vi "Joystick and Camera.vi"() -> ()   [LabVIEW 2021]
uses:
  Classes/Controller/Camera/Machine Vision.ctl
  Classes/Controller/Camera/Image processing.ctl
  Classes/Controller/Camera/Camera settings.ctl
  Classes/Controller/Camera/Material.ctl
  Classes/Controller/I-O/I-O.lvclass
  Classes/Controller/Camera/Camera.lvclass
  Classes/Controller/Controller.lvclass
  Classes/Controller/Motion/A3200/A3200.lvclass
  Classes/Controller/Motion/Motion.lvclass
  <vilib>/vision/driver/NI_Vision_Acquisition_Software.lvlib
panel:
  out "Move by":dbl[](array[numeric])
  in  "Autofiducial":bool
  in  "Screen Grab":bool
  in  "Focus step size":dbl format="%#_13g"
  in  "number of focus steps":i32
  out "Radius (Real-World)":dbl
  out "error out":errorcluster
  in  "Find fiducial center":bool
  out "Average Strength":dbl
  in  "Focus":bool
  in  "Material":T1
  in  "Override presets":bool
  in  "Camera settings":T2={"Gamma"=1.6, "Gain"=0, "Sharpness"=0, "Contrast"=0.0, "Exposure"=0.0078125} {"Exposure" min=0.000244140625 max=0.5 scale=0.0002..0.5; "Contrast" min=0.0 max=1.0 scale=0.0..1.0; "Sharpness" min=0 max=2 step=1 scale=0.0..2.0; "Gain" min=0 max=100 step=1 scale=0.0..100.0; "Gamma" min=0.01 max=10.0 scale=0.01..10.0}
  in  "Image processing":T3={"Brightness"=128.0, "Contrast"=45.0, "Gamma"=1.0471123} {"Brightness" scale=0.0..400.0; "Contrast" scale=0.0..90.0; "Gamma" scale=0.005..5.0}
  out "XYZTheta Out":dbl[](array[numeric])
  in  "Machine Vision":T4
  in  "Move 10cm Right":bool
  in  "Move 10cm Backward":bool
  in  "Move 10cm Forward":bool
  in  "Move 10cm Left":bool
  in  "Record Measurement":bool=TRUE
  in  "Dismount Silicon Tray":bool
  in  "Secure Silicon Tray":bool
  in  "Z Go":bool
  in  "Position":dbl
  in  "XYZTheta":dbl[](array[numeric])
  in  "Go":bool
  in  "Joystick":bool
  out "Sum":dbl[](array[numeric]) format="%#.6g"
  out "Gantry":dbl[](array[numeric]) format="%#.6g"
  in  "Stop":bool
  out "Image":T5(plugin-control)
  out "Camera":dbl[](array[numeric])
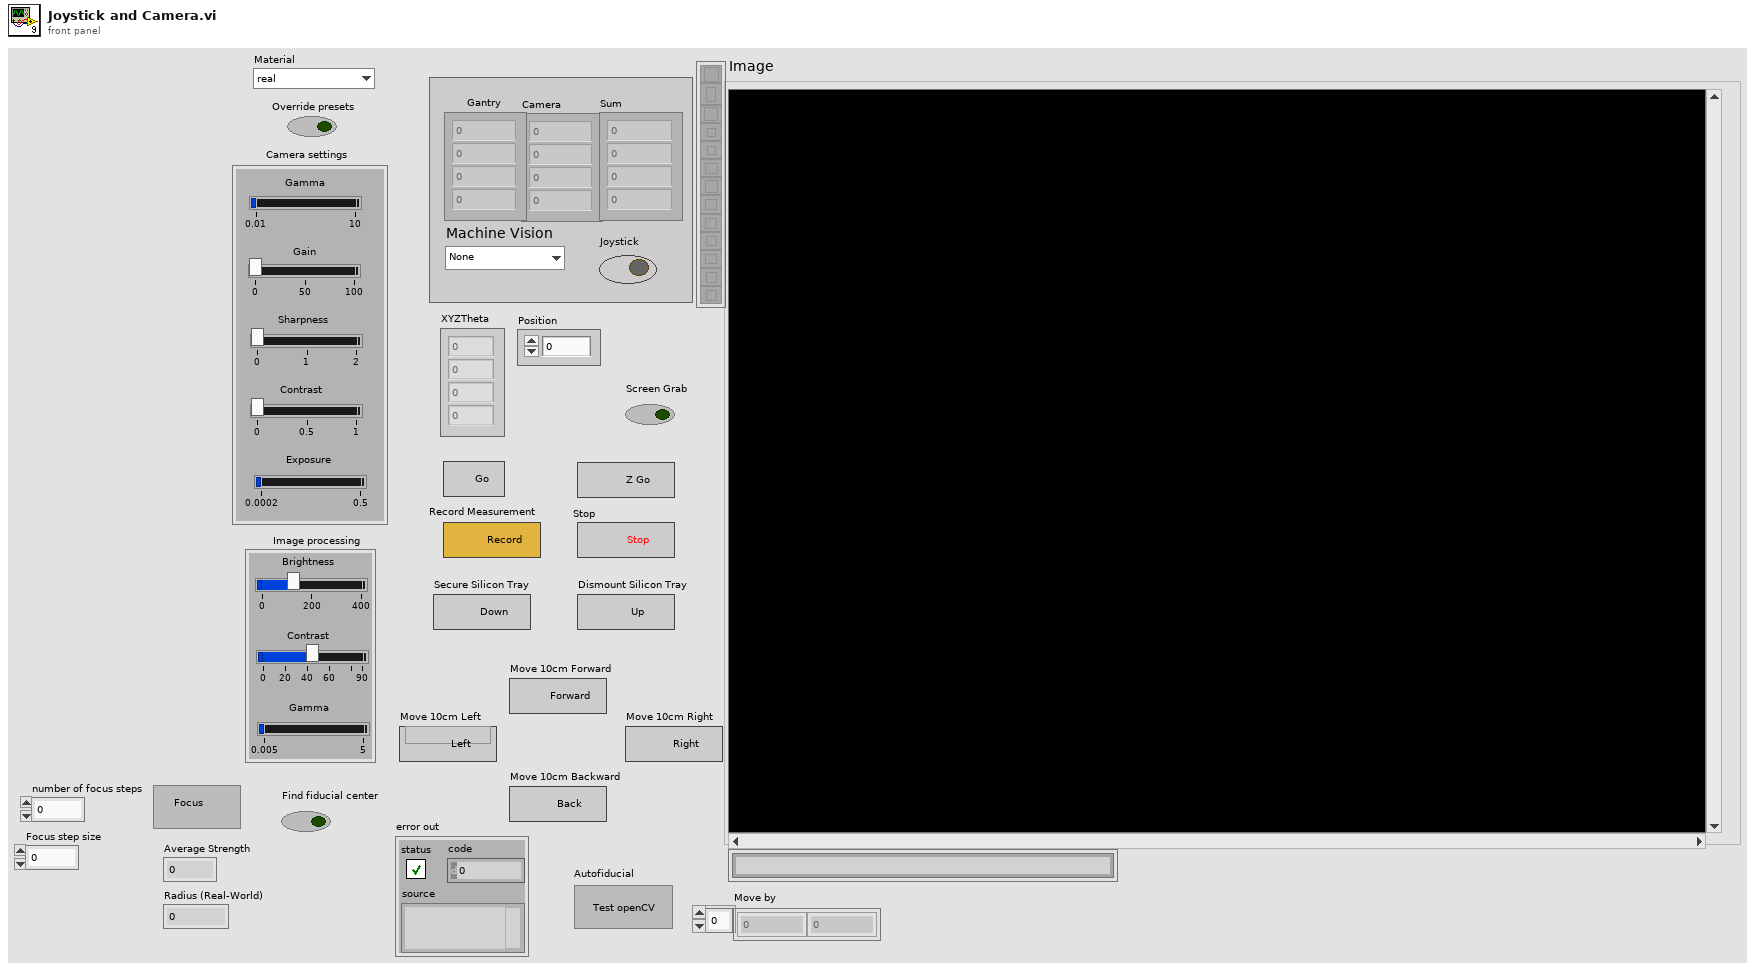
[diagram p1: front panel]
types:
  T1 = typedef "Camera.lvclass/Material.ctl" = enum16{"real", "dummy", "PETG"}
  T2 = typedef "Camera.lvclass/Camera settings.ctl" = cluster{"Gamma":dbl, "Gain":i64, "Sharpness":i64, "Contrast":dbl, "Exposure":dbl}
  T3 = typedef "Camera.lvclass/Image processing.ctl" = cluster{"Brightness":sgl, "Contrast":sgl, "Gamma":sgl}
  T4 = typedef "Camera.lvclass/Machine Vision.ctl" = enum16{"None", "Tray Fiducials", "HPK Silicon", "100um dot", "Hexaboard", "Corner (TL, BR)", "Corner (BL, TR)", "BP gold pad 1", "BP gold pad 2", "BP gold pad 3", "dummy sensor CH2", "dummy sensor CH7", "dummy sensor CH191", "dummy sensor CH197", "sensor circle", "sensor cross"}
  T5 = typedef "IMAQ Image.ctl" = refnum<image>
  T6 = enum16{"open", "replace", "create", "open or create", "replace or create", "replace or create with confirmation"}
  T7 = typedef "Controller.lvclass/Controllers.ctl" = cluster{"I-O.lvclass":refnum<class "I-O.lvclass">, "Gantry":refnum<k24>, "Dispenser":refnum<visa-resource-name>}
  T8 = typedef "I-O.lvclass/Pin Map.ctl" = cluster{"Region Valves":i32[], "Extra Valves":dbl[][][], "Tool Primary Valve":i32, "Tool Secondary Valve":i32, "Region Sensors":i32[], "Extra Sensors":dbl[][][], "Tool Primary Sensor":dbl, "Tool Secondary Sensor":dbl, "Compression Sensor":dbl, "5V":i32, "Dispenser Sensor":dbl}
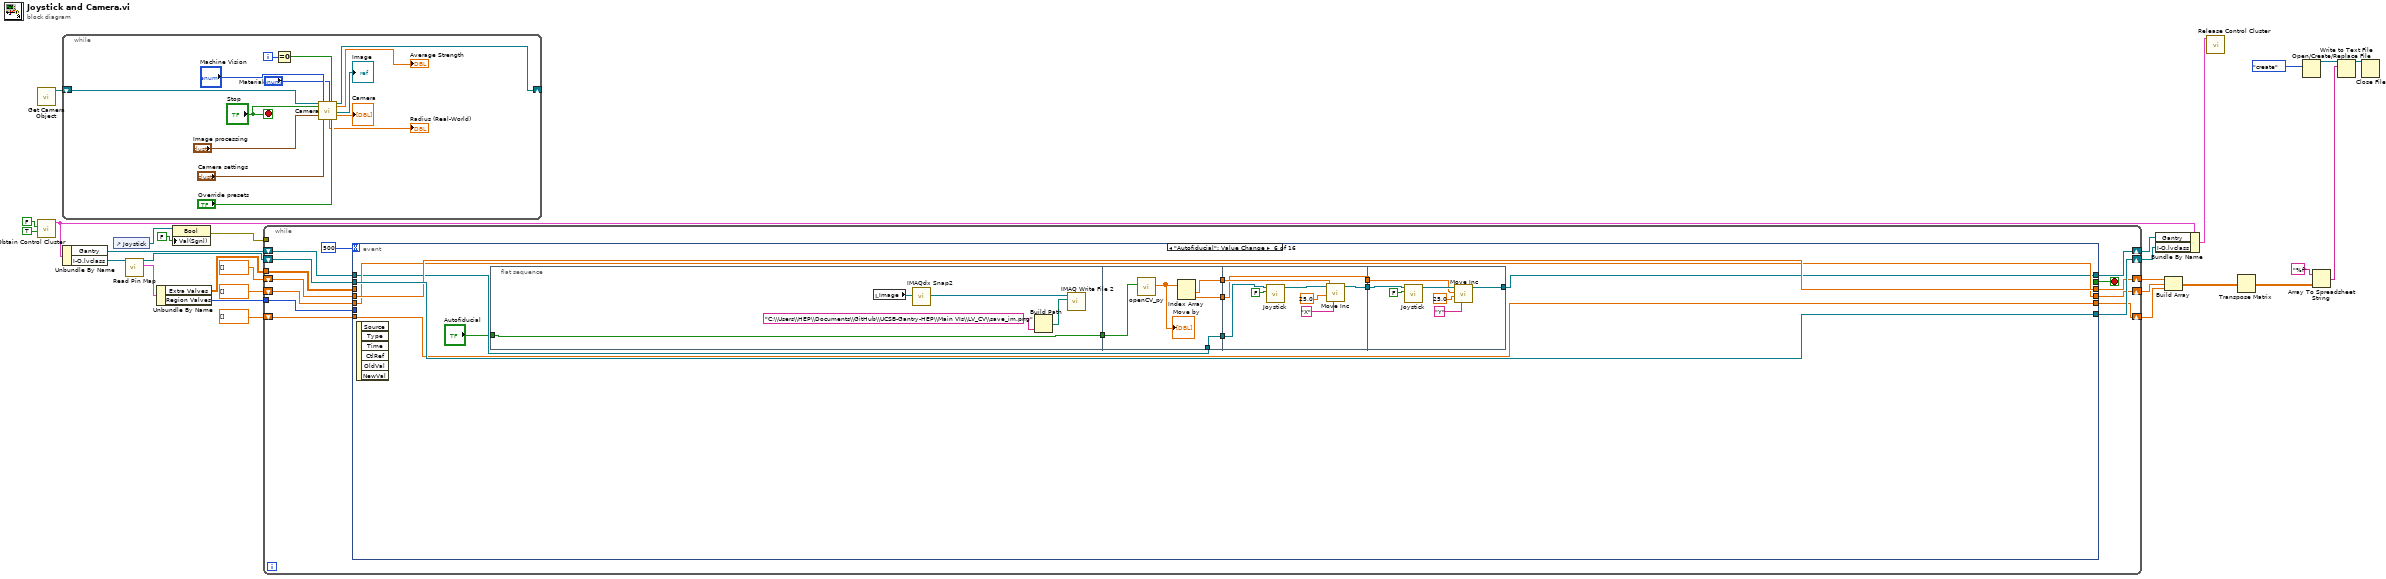
[diagram p0: block diagram]
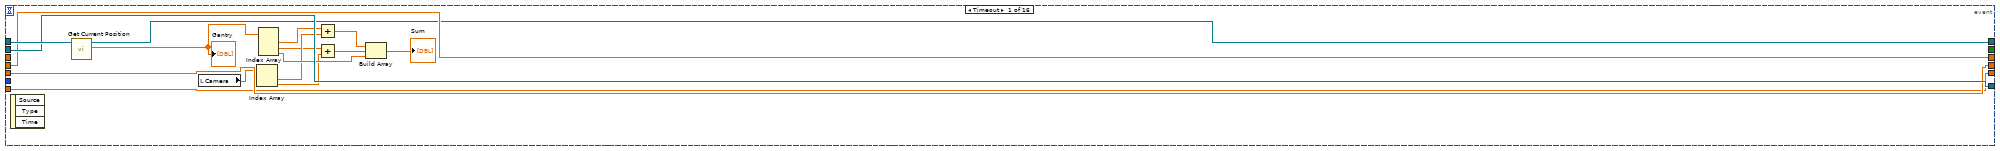
[diagram p2: hidden frame]
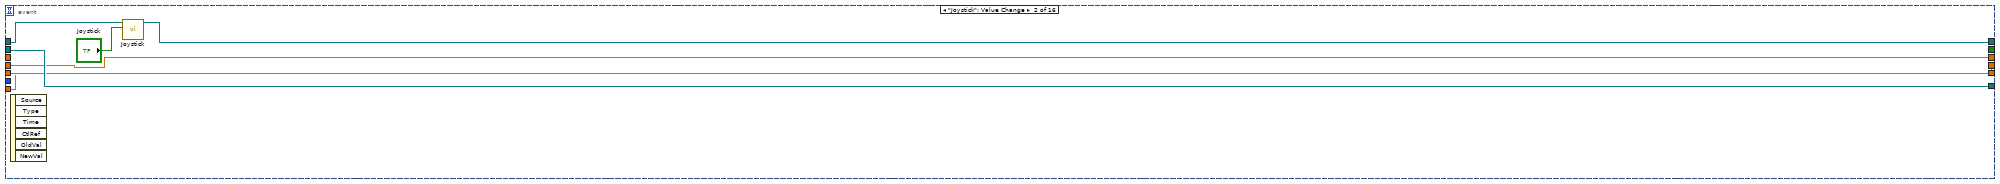
[diagram p3: hidden frame]
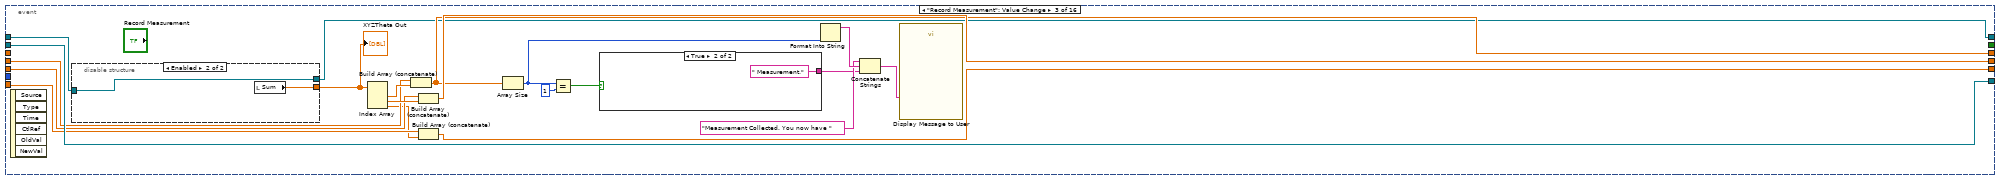
[diagram p4: hidden frame]
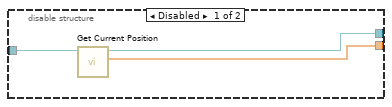
[diagram p5: hidden frame]
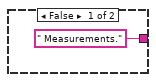
[diagram p6: hidden frame]
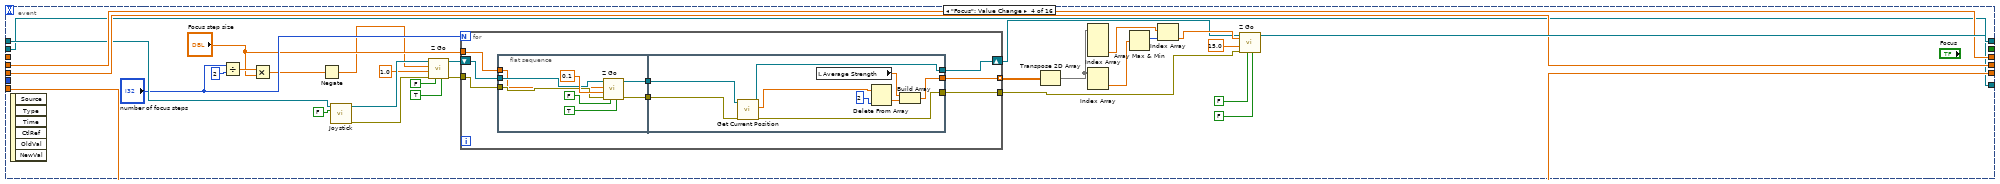
[diagram p7: hidden frame]
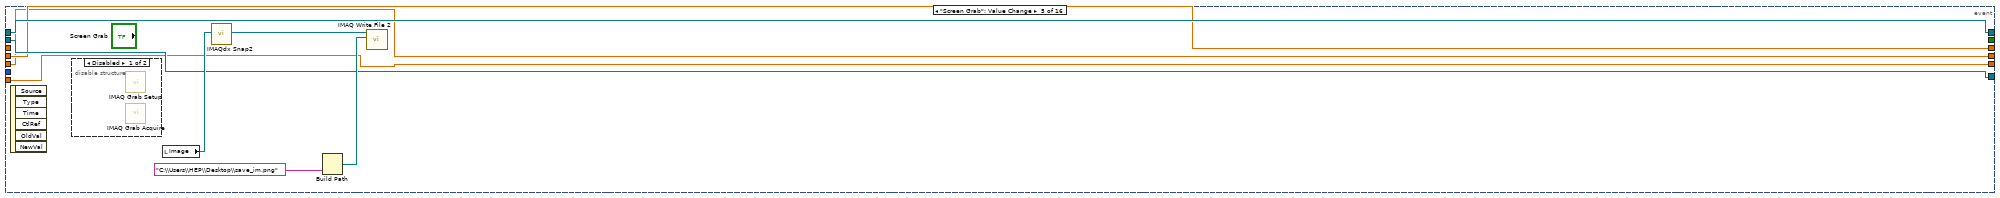
[diagram p8: hidden frame]
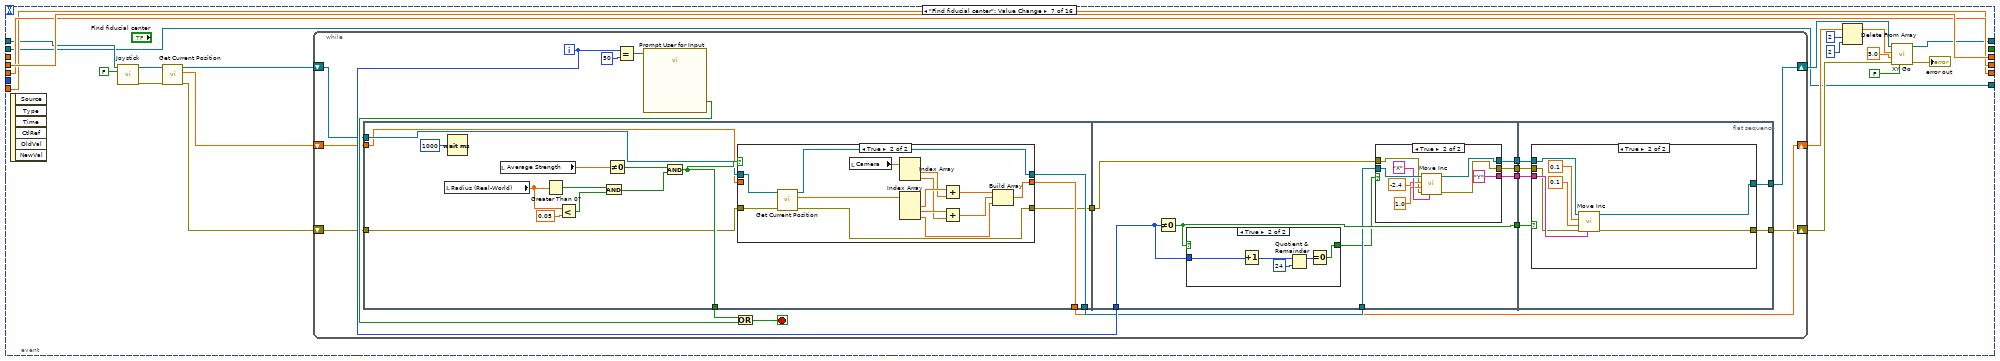
[diagram p10: hidden frame]
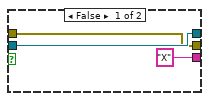
[diagram p13: hidden frame]
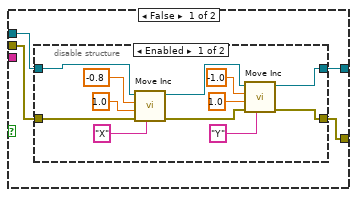
[diagram p14: hidden frame]
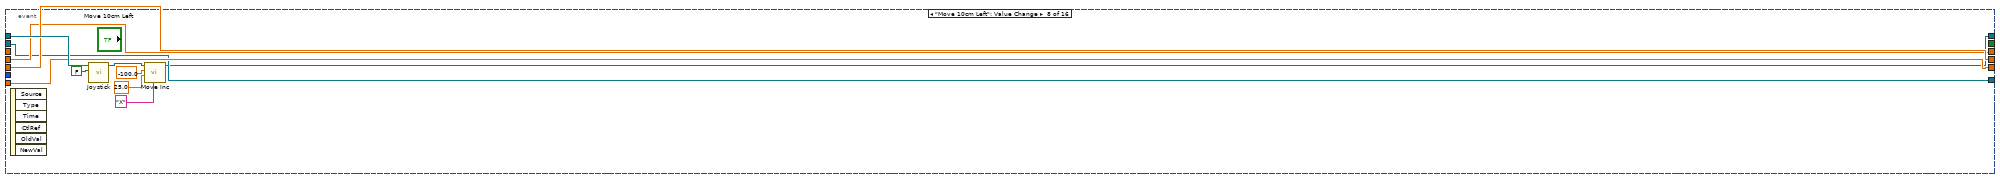
[diagram p16: hidden frame]
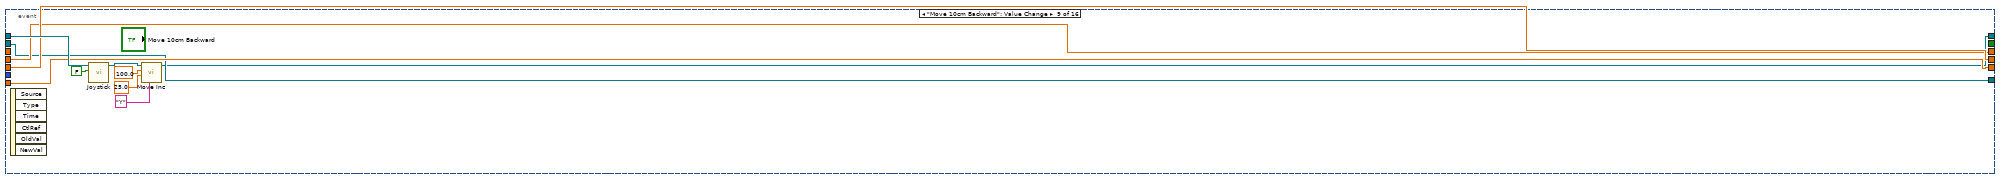
[diagram p17: hidden frame]
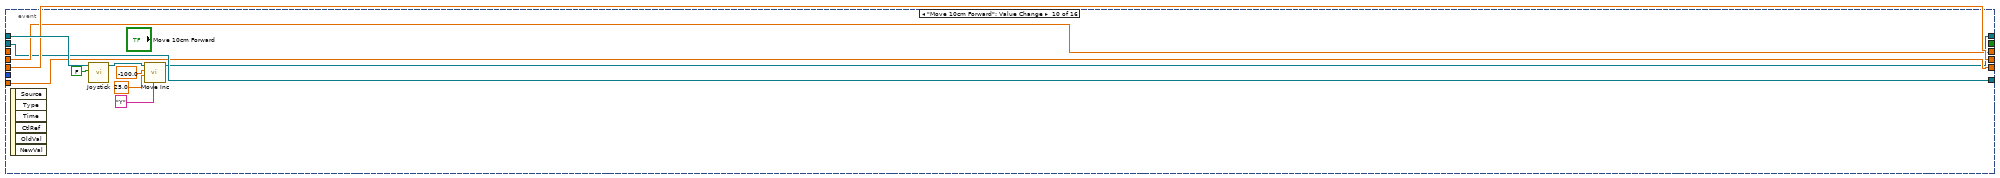
[diagram p18: hidden frame]
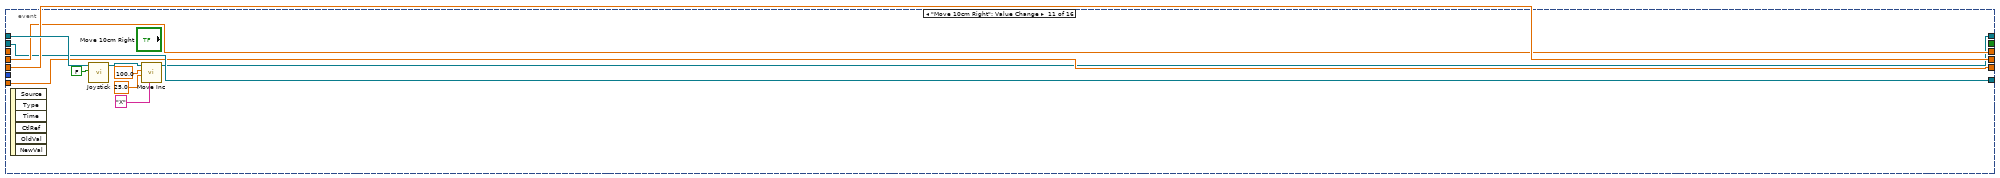
[diagram p19: hidden frame]
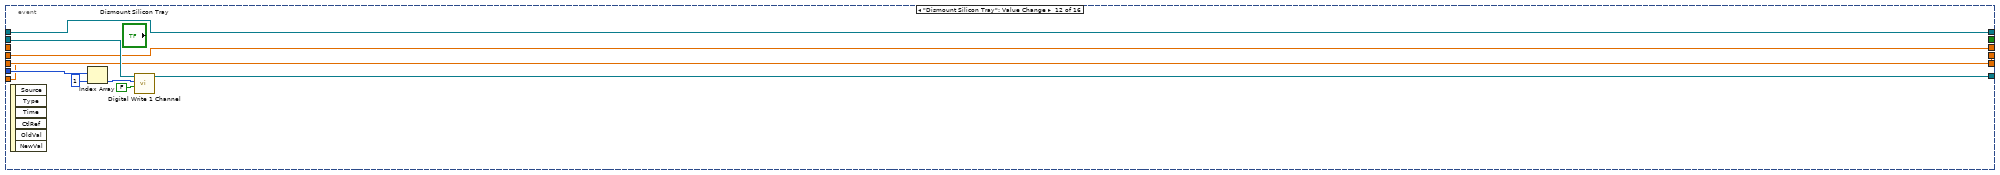
[diagram p20: hidden frame]
diagram:
  n1 = call "Get Camera Object.vi"() -> ("Camera out"=w23:refnum<class "Camera.lvclass">)  [unwired: 10 in, 1 out]
  n2 = call "Obtain Control Cluster.vi"("I/O"=TRUE, "Dispense"=FALSE) -> ("Control Out"=w1:T7)  [unwired: 9 in]
  n3 = while {
    shift-right: [w42] -> _
    shift-left: w23 -> [w43]
    i -> [w34]
    stop <- "Stop" stop-if-true
    n4 = Equal To 0?(x=w34) -> (x = 0?=w33:bool)
    n5 = call "Camera.vi"("Camera in"=w43, "Stop"="Stop", "BCG Image Processing"="Image processing", "Machine Vision"="Machine Vision", "Camera settings"="Camera settings", "Material"="Material", "Loop 0"=w33, "Override presets"="Override presets") -> ("Radius (Real-World)"=→"Radius (Real-World)":dbl, "Camera out"=w42:refnum<class "Camera.lvclass">, "Average Strength"=→"Average Strength":dbl, "Image"=→"Image":T5, "Camera"=→"Camera":dbl[])  [unwired: 6 in, 1 out]
  }
  n6 = Unbundle By Name(w1) -> ("Gantry"=w24:refnum<k24>, "I-O.lvclass"=w22:refnum<class "I-O.lvclass">)
  n7 = control-ref of="Joystick"() -> (w28:refnum<vi>)
  n8 = call-dynamic "Read Pin Map.vi"("I-O in"=w22) -> ("Pin Map 2"=w20:T8, "I-O out"=w21:refnum<class "I-O.lvclass">)  [unwired: 8 in, 1 out]
  n9 = Unbundle By Name(w20) -> ("Extra Valves"=w18:dbl[][][], "Region Valves"=w19:i32[])
  n10 = property class="Bool"(reference=w28, "Val(Sgnl)"=FALSE ("Value (Signaling)")) -> (error out=w27:errorcluster)  [unwired: 1 in, 1 out]
  n11 = while {
    shift-right: [w44] -> w4
    shift-left: w24 -> [w55]
    tunnel: w27 -> [_]
    shift-right: [w53] -> w3
    shift-left: w21 -> [w54]
    tunnel: w19 -> [w52]
    tunnel: w18 -> [w51]
    shift-right: [w46] -> w6
    shift-left: dbl[] [] -> [w50]
    shift-right: [w48] -> w7
    shift-left: dbl[] [] -> [w49]
    shift-right: [w45] -> w8
    shift-left: dbl[] [] -> [w47]
    stop <- w56 stop-if-true
    n12 = event shown="[5] \"Autofiducial\": Value Change" {
      selector: _ -> [_ _ _ _ _ _ _ _ _ _ _ _ _ _ _ _]
      dyn-events: _ -> [_ _ _ _ _ _ _ _ _ _ _ _ _ _ _ _]
      timeout: 500 -> [_ _ _ _ _ _ _ _ _ _ _ _ _ _ _ _]
      tunnel: [_ _ _ _ _ _ _ _ _ _ _ _ _ _ _ TRUE] -> w56
      tunnel: w55 -> [w73 w80 w83 w124 w168 w180 w228 w347 w358 w369 w380 w382 w392 w409 w428 w436]
      tunnel: w54 -> [w72 w78 w100 w108 w167 w185 w211 w342 w354 w366 w377 w389 w401 w406 w425 w434]
      tunnel: [w72 w78 w100 w108 w167 w185 w211 w342 w354 w366 w377 w386 w396 w406 w425 w434] -> w53
      tunnel: w52 -> [_ _ _ _ _ _ _ _ _ _ _ w391 w400 _ _ _]
      tunnel: w51 -> [_ _ _ _ _ _ _ _ _ _ _ _ _ _ _ _]
      tunnel: w50 -> [w71 w77 w87 w127 w165 w183 w230 w345 w357 w368 w379 w385 w395 w405 w424 w433]
      tunnel: [w71 w77 w91 w127 w165 w183 w230 w345 w357 w368 w379 w385 w395 w405 w424 w433] -> w46
      tunnel: w49 -> [w70 w76 w88 w128 w166 w184 w231 w344 w356 w367 w378 w384 w394 w404 w423 w432]
      tunnel: [w70 w76 w90 w128 w166 w184 w231 w344 w356 w367 w378 w384 w394 w404 w423 w432] -> w48
      tunnel: w47 -> [w69 w75 w86 w126 w164 w182 w229 w343 w355 w365 w376 w383 w393 w403 w422 w431]
      tunnel: [w69 w75 w84 w126 w164 w182 w229 w343 w355 w365 w376 w383 w393 w403 w422 w431] -> w45
      tunnel: [w68 w74 w81 w129 w168 w179 w225 w341 w350 w360 w372 w382 w392 w402 w421 w429] -> w44
      event Timeout {
        n13 = event-data() -> ()  [unwired: 1 in, 3 out]
        n14 = call "Get Current Position.vi"("Gantry In"=w73) -> ("XYZTheta Out"=w65:dbl[], "Gantry Out"=w68:refnum<k24>)  [unwired: 8 in, 1 out]
        "Gantry" <- w65
        n15 = local read "Camera"() -> (w62:dbl[])
        n16 = Index Array(array=w62) -> (element #1=w61:dbl, element #2=w58:dbl)  [unwired: 2 in]
        n17 = Index Array(array=w65) -> (element #1=w63:dbl, element #2=w59:dbl, element #3=w66:dbl)  [unwired: 3 in]
        n18 = Add(x=w63, y=w61) -> (x+y=w64:dbl)
        n19 = Add(x=w59, y=w58) -> (x+y=w60:dbl)
        n20 = Build Array(w64, w60, w66) -> (→"Sum":dbl[])
      }
      event "Joystick": Value Change {
        n21 = event-data() -> ()  [unwired: 1 in, 6 out]
        n22 = call "Joystick.vi"("Joystick"="Joystick", "Gantry In"=w80) -> ("Gantry Out"=w74:refnum<k24>)  [unwired: 8 in, 1 out]
      }
      event "Record Measurement": Value Change {
        n23 = event-data() -> ()  [unwired: 1 in, 6 out]
        n24 = disable-structure shown="Enabled" {
          disable-tunnel: [w102 w104] -> w82
          disable-tunnel: w83 -> [w103 w105]
          disable-tunnel: [w101 w105] -> w81
          frame Disabled {
            n25 = call "Get Current Position.vi"("Gantry In"=w103) -> ("XYZTheta Out"=w102:dbl[], "Gantry Out"=w101:refnum<k24>)  [unwired: 8 in, 1 out]
          }
          frame Enabled {
            n26 = local read "Sum"() -> (w104:dbl[])
          }
        }
        "XYZTheta Out" <- w82
        n27 = Index Array(array=w82) -> (element #1=w99:dbl, element #2=w89:dbl, element #3=w85:dbl)  [unwired: 3 in]
        n28 = Build Array (concatenate) "Build Array"(w88, w99) -> (w90:dbl[])
        n29 = Build Array (concatenate)(w87, w89) -> (w91:dbl[])
        n30 = Build Array (concatenate)(w86, w85) -> (w84:dbl[])
        n31 = Array Size(array=w90) -> (size(s)=w94:i32)
        n32 = Equal?(x=w94, y=1) -> (x = y?=w93:bool)
        n33 = case shown="True" w93 {
          tunnel: [" Measurements." " Measurement."] -> w92
          frame False {
          }
          frame True {
          }
        }
        n34 = Format Into String(w94) -> (resulting string=w98:string)  [unwired: 3 in, 1 out]
        n35 = Concatenate Strings("Measurement Collected. You now have ", w98, w92) -> (w96:string)
        n36 = call "Display Message to User"("Message"=w96) -> ()  [unwired: 9 in, 2 out]
      }
      event "Focus": Value Change {
        n37 = event-data() -> ()  [unwired: 1 in, 6 out]
        n38 = Divide(x="number of focus steps", y=2) -> (x/y=w121:dbl)
        n39 = Multiply(x=w121, y="Focus step size") -> (x*y=w119:dbl)
        n40 = Negate(x=w119) -> (-x=w114:dbl)
        n41 = call "Joystick.vi"("Joystick"=FALSE, "Gantry In"=w124) -> ("error out"=w115:errorcluster, "Gantry Out"=w118:refnum<k24>)  [unwired: 8 in]
        n42 = call "Z Go.vi"("Increment"=TRUE, "Return Immediately"=FALSE ("Increment"), "error in (no error)"=w115, "Speed In"=1.0 ("Speed"), "Position In"=w114, "Gantry In"=w118) -> ("error out"=w116:errorcluster, "Gantry Out"=w117:refnum<k24>)  [unwired: 2 in, 2 out]
        n43 = for {
          N: "number of focus steps" -> [_]
          tunnel: [w143] -> w137 mode=indexing
          tunnel: w116 -> [w142]
          tunnel: [w140] -> w130
          shift-right: [w144] -> w131
          shift-left: w117 -> [w146]
          tunnel: "Focus step size" -> [w139]
          n44 = flat-sequence {
            tunnel: w146 -> [w153]
            tunnel: [w152] -> w145
            tunnel: w142 -> [w151]
            tunnel: [w150] -> w141
            tunnel: w139 -> [w149]
            tunnel: w145 -> [w163]
            tunnel: [w162] -> w144
            tunnel: [w161] -> w143
            tunnel: w141 -> [w157]
            tunnel: [w156] -> w140
            frame #0 {
              n45 = call "Z Go.vi"("Increment"=TRUE, "Return Immediately"=FALSE ("Increment"), "error in (no error)"=w151, "Speed In"=0.1 ("Speed"), "Position In"=w149, "Gantry In"=w153) -> ("error out"=w150:errorcluster, "Gantry Out"=w152:refnum<k24>)  [unwired: 2 in, 2 out]
            }
            frame #1 {
              n46 = call "Get Current Position.vi"("error in (no error)"=w157, "Gantry In"=w163) -> ("error out"=w156:errorcluster, "XYZTheta Out"=w160:dbl[], "Gantry Out"=w162:refnum<k24>)  [unwired: 7 in]
              n47 = local read "Average Strength"() -> (w155:dbl)
              n48 = Delete From Array(array=w160, index=2) -> (deleted portion=w158:dbl)  [unwired: 1 in, 1 out]
              n49 = Build Array(w155, w158) -> (w161:dbl[])
            }
          }
        }
        n50 = Transpose 2D Array(2D array=w137) -> (transposed array=w136:dbl[][])
        n51 = Index Array(array=w136) -> (element #2=w135:dbl[])  [unwired: 4 in, 1 out]
        n52 = Index Array(array=w136) -> (element=w138:dbl[])  [unwired: 2 in]
        n53 = Array Max & Min(array=w138) -> (max index (indices)=w134:i32)  [unwired: 3 out]
        n54 = Index Array(array=w135, index=w134) -> (element=w133:dbl)
        n55 = call "Z Go.vi"("Increment"=FALSE, "Return Immediately"=FALSE ("Increment"), "error in (no error)"=w130, "Speed In"=15.0 ("Speed"), "Position In"=w133, "Gantry In"=w131) -> ("Gantry Out"=w129:refnum<k24>)  [unwired: 2 in, 3 out]
      }
      event "Screen Grab": Value Change {
        n56 = event-data() -> ()  [unwired: 1 in, 6 out]
        n57 = disable-structure shown="Disabled" {
          frame Disabled {
            n58 = call <vilib>:"IMAQ Grab Setup.vi"() -> ()  [unwired: 10 in, 2 out]
            n59 = call <vilib>:"IMAQ Grab Acquire.vi"() -> ()  [unwired: 8 in, 4 out]
          }
          frame Enabled {
          }
        }
        n60 = local read "Image"() -> (w172:T5)
        n61 = call <vilib>:"IMAQdx Snap2.vi"("Image In"=w172) -> ("Image Out"=w171:T5)  [unwired: 8 in, 2 out]
        n62 = Build Path(name or relative path="C:\\Users\\HEP\\Desktop\\save_im.png") -> (appended path=w170:path)  [unwired: 1 in]
        n63 = call-poly "IMAQ Write File 2"("File Path"=w170, "Image"=w171) -> ()  [unwired: 8 in, 2 out]
      }
      event "Autofiducial": Value Change {
        n64 = event-data() -> ()  [unwired: 1 in, 6 out]
        n65 = flat-sequence {
          tunnel: [w186] -> w181
          tunnel: "Autofiducial" -> [w186]
          tunnel: w181 -> [w195]
          tunnel: w180 -> [w194]
          tunnel: [w194] -> w177
          tunnel: [w192] -> w175
          tunnel: [w191] -> w173
          tunnel: w177 -> [w199]
          tunnel: [w198] -> w176
          tunnel: w175 -> [w197]
          tunnel: [w196] -> w174
          tunnel: w173 -> [w196]
          tunnel: [w205] -> w179
          tunnel: w176 -> [w206]
          tunnel: w174 -> [w204]
          frame #0 {
            n66 = local read "Image"() -> (w190:T5)
            n67 = call <vilib>:"IMAQdx Snap2.vi"("Image In"=w190) -> ("Image Out"=w189:T5)  [unwired: 8 in, 2 out]
            n68 = Build Path(name or relative path="C:\\Users\\HEP\\Documents\\GitHub\\UCSB-Gantry-HEP\\Main VIs\\LV_CV\\save_im.png") -> (appended path=w188:path)  [unwired: 1 in]
            n69 = call-poly "IMAQ Write File 2"("File Path"=w188, "Image"=w189) -> ()  [unwired: 8 in, 2 out]
          }
          frame #1 {
            n70 = call "openCV_py.vi"("Run PY"=w195) -> ("Move by"=w193:dbl[])  [unwired: 10 in]
            "Move by" <- w193
            n71 = Index Array(array=w193) -> (element #1=w192:dbl, element #2=w191:dbl)  [unwired: 2 in]
          }
          frame #2 {
            n72 = call "Joystick.vi"("Joystick"=FALSE, "Gantry In"=w199) -> ("Gantry Out"=w200:refnum<k24>)  [unwired: 8 in, 1 out]
            n73 = call "Move Inc.vi"("Axis"="X", "Speed"=25.0, "Distance"=w197, "Gantry In"=w200) -> ("Gantry Out"=w198:refnum<k24>)  [unwired: 6 in, 1 out]
          }
          frame #3 {
            n74 = call "Joystick.vi"("Joystick"=FALSE, "Gantry In"=w206) -> ("Gantry Out"=w207:refnum<k24>)  [unwired: 8 in, 1 out]
            n75 = call "Move Inc.vi"("Axis"="Y", "Speed"=25.0, "Distance"=w204, "Gantry In"=w207) -> ("Gantry Out"=w205:refnum<k24>)  [unwired: 6 in, 1 out]
          }
        }
      }
      event "Find fiducial center": Value Change {
        n76 = event-data() -> ()  [unwired: 1 in, 6 out]
        n77 = call "Joystick.vi"("Joystick"=FALSE, "Gantry In"=w228) -> ("error out"=w217:errorcluster, "Gantry Out"=w219:refnum<k24>)  [unwired: 8 in]
        n78 = call "Get Current Position.vi"("error in (no error)"=w217, "Gantry In"=w219) -> ("error out"=w216:errorcluster, "XYZTheta Out"=w214:dbl[], "Gantry Out"=w218:refnum<k24>)  [unwired: 7 in]
        n79 = while {
          shift-right: [w248] -> w226
          shift-left: w218 -> [w237]
          shift-right: [w249] -> w224
          shift-left: w216 -> [w234]
          shift-right: [w232] -> w213
          shift-left: w214 -> [w235]
          i -> [w243]
          stop <- w241 stop-if-true
          n80 = flat-sequence {
            tunnel: [w261] -> w238
            tunnel: [w260] -> w232
            tunnel: w237 -> [w259]
            tunnel: [w258] -> w236
            tunnel: w235 -> [w257]
            tunnel: w234 -> [w256]
            tunnel: [w255] -> w233
            tunnel: w243 -> [w289]
            tunnel: [w288] -> w247
            tunnel: [w287] -> w246
            tunnel: w236 -> [w286]
            tunnel: [w285] -> w245
            tunnel: [w284] -> w244
            tunnel: w233 -> [w282]
            tunnel: [w310] -> w248
            tunnel: [w311] -> w249
            tunnel: w247 -> [w312]
            tunnel: w246 -> [w309]
            tunnel: w245 -> [w308]
            tunnel: w244 -> [w307]
            frame #0 {
              n81 = local read "Radius (Real-World)"() -> (w251:dbl)
              n82 = Wait (ms)(milliseconds to wait=u32 1000) -> ()  [unwired: 1 out]
              n83 = local read "Average Strength"() -> (w264:dbl)
              n84 = Greater Than 0?(x=w251) -> (x > 0?=w253:bool)
              n85 = Less?(x=w251, y=0.05) -> (x < y?=w252:bool)
              n86 = And(x=w253, y=w252) -> (x .and. y?=w262:bool)
              n87 = Not Equal To 0?(x=w264) -> (x != 0?=w263:bool)
              n88 = And(x=w263, y=w262) -> (x .and. y?=w261:bool)
              n89 = case shown="True" w261 {
                tunnel: [w266 w270] -> w260
                tunnel: w259 -> [w267 w281]
                tunnel: [w267 w280] -> w258
                tunnel: w257 -> [w266 _]
                tunnel: w256 -> [w265 w269]
                tunnel: [w265 w268] -> w255
                frame False {
                }
                frame True {
                  n90 = call "Get Current Position.vi"("error in (no error)"=w269, "Gantry In"=w281) -> ("error out"=w268:errorcluster, "XYZTheta Out"=w279:dbl[], "Gantry Out"=w280:refnum<k24>)  [unwired: 7 in]
                  n91 = local read "Camera"() -> (w277:dbl[])
                  n92 = Index Array(array=w277) -> (element #1=w274:dbl, element #2=w273:dbl)  [unwired: 2 in]
                  n93 = Index Array(array=w279) -> (element #1=w278:dbl, element #2=w275:dbl, element #3=w276:dbl)  [unwired: 3 in]
                  n94 = Add(x=w278, y=w274) -> (x+y=w272:dbl)
                  n95 = Add(x=w275, y=w273) -> (x+y=w271:dbl)
                  n96 = Build Array(w272, w271, w276) -> (w270:dbl[])
                }
              }
            }
            frame #1 {
              n97 = Not Equal To 0?(x=w289) -> (x != 0?=w287:bool)
              n98 = case shown="True" w287 {
                selector: w287 -> [w290 _]
                tunnel: [w290 w294] -> w283
                tunnel: w289 -> [_ w292]
                frame False {
                }
                frame True {
                  n99 = Increment(x=w292) -> (x+1=w291:i32)
                  n100 = Quotient & Remainder(x=w291, y=24) -> (x-y*floor(x/y)=w293:i32)  [unwired: 1 out]
                  n101 = Equal To 0?(x=w293) -> (x = 0?=w294:bool)
                }
              }
              n102 = case shown="True" w283 {
                tunnel: ["X" ("Axis") "Y" ("Axis")] -> w288
                tunnel: w286 -> [w297 w305]
                tunnel: [w297 w304] -> w285
                tunnel: [w296 w300] -> w284
                tunnel: w282 -> [w296 w299]
                frame False {
                }
                frame True {
                  n103 = call "Move Inc.vi"("Axis"="X", "error in (no error)"=w299, "Speed"=1.0, "Distance"=-2.4, "Gantry In"=w305) -> ("error out"=w300:errorcluster, "Gantry Out"=w304:refnum<k24>)  [unwired: 5 in]
                }
              }
            }
            frame #2 {
              n104 = case shown="True" w309 {
                tunnel: w312 -> [_ w337]
                tunnel: w307 -> [w313 w336]
                tunnel: w308 -> [w316 w334]
                tunnel: [w314 w333] -> w311
                tunnel: [w315 w332] -> w310
                frame False {
                  n105 = disable-structure shown="Enabled" {
                    disable-tunnel: w316 -> [w328 w330]
                    disable-tunnel: [w326 w330] -> w315
                    disable-tunnel: [w325 w329] -> w314
                    disable-tunnel: w313 -> [w323 w329]
                    frame Enabled {
                      n106 = call "Move Inc.vi"("Axis"="X", "error in (no error)"=w323, "Speed"=1.0, "Distance"=-0.8, "Gantry In"=w328) -> ("error out"=w324:errorcluster, "Gantry Out"=w327:refnum<k24>)  [unwired: 5 in]
                      n107 = call "Move Inc.vi"("Axis"="Y", "error in (no error)"=w324, "Speed"=1.0, "Distance"=-1.0, "Gantry In"=w327) -> ("error out"=w325:errorcluster, "Gantry Out"=w326:refnum<k24>)  [unwired: 5 in]
                    }
                    frame Disabled {
                    }
                  }
                }
                frame True {
                  n108 = call "Move Inc.vi"("Axis"=w337, "error in (no error)"=w336, "Speed"=0.1, "Distance"=0.1, "Gantry In"=w334) -> ("error out"=w333:errorcluster, "Gantry Out"=w332:refnum<k24>)  [unwired: 5 in]
                }
              }
            }
          }
          n109 = Equal?(x=w243, y=50) -> (x = y?=w240:bool)
          n110 = call "Prompt User for Input"("Enable"=w240) -> ("OK"=w239:bool)  [unwired: 17 in, 1 out]
          n111 = Or(x=w238, y=w239) -> (x .or. y?=w241:bool)
        }
        n112 = Delete From Array(array=w213, length=2, index=2) -> (array with subset deleted=w221:dbl[])  [unwired: 1 out]
        n113 = call "XY Go.vi"("return immediately"=FALSE, "error in (no error)"=w224, "Speed"=5.0, "XY In"=w221, "Gantry In"=w226) -> ("error out"=→"error out":errorcluster, "Gantry Out"=w225:refnum<k24>)  [unwired: 4 in, 1 out]
      }
      event "Move 10cm Left": Value Change {
        n114 = event-data() -> ()  [unwired: 1 in, 6 out]
        n115 = call "Joystick.vi"("Joystick"=FALSE, "Gantry In"=w347) -> ("Gantry Out"=w338:refnum<k24>)  [unwired: 8 in, 1 out]
        n116 = call "Move Inc.vi"("Axis"="X", "Speed"=25.0, "Distance"=-100.0, "Gantry In"=w338) -> ("Gantry Out"=w341:refnum<k24>)  [unwired: 6 in, 1 out]
      }
      event "Move 10cm Backward": Value Change {
        n117 = event-data() -> ()  [unwired: 1 in, 6 out]
        n118 = call "Joystick.vi"("Joystick"=FALSE, "Gantry In"=w358) -> ("Gantry Out"=w349:refnum<k24>)  [unwired: 8 in, 1 out]
        n119 = call "Move Inc.vi"("Axis"="Y", "Speed"=25.0, "Distance"=100.0, "Gantry In"=w349) -> ("Gantry Out"=w350:refnum<k24>)  [unwired: 6 in, 1 out]
      }
      event "Move 10cm Forward": Value Change {
        n120 = event-data() -> ()  [unwired: 1 in, 6 out]
        n121 = call "Joystick.vi"("Joystick"=FALSE, "Gantry In"=w369) -> ("Gantry Out"=w361:refnum<k24>)  [unwired: 8 in, 1 out]
        n122 = call "Move Inc.vi"("Axis"="Y", "Speed"=25.0, "Distance"=-100.0, "Gantry In"=w361) -> ("Gantry Out"=w360:refnum<k24>)  [unwired: 6 in, 1 out]
      }
      event "Move 10cm Right": Value Change {
        n123 = event-data() -> ()  [unwired: 1 in, 6 out]
        n124 = call "Joystick.vi"("Joystick"=FALSE, "Gantry In"=w380) -> ("Gantry Out"=w371:refnum<k24>)  [unwired: 8 in, 1 out]
        n125 = call "Move Inc.vi"("Axis"="X", "Speed"=25.0, "Distance"=100.0, "Gantry In"=w371) -> ("Gantry Out"=w372:refnum<k24>)  [unwired: 6 in, 1 out]
      }
      event "Dismount Silicon Tray": Value Change {
        n126 = event-data() -> ()  [unwired: 1 in, 6 out]
        n127 = Index Array(array=w391, index=1) -> (element=w388:i32)
        n128 = call-dynamic "Digital Write 1 Channel.vi"("Value"=FALSE, "Channel"=w388, "I-O.lvclass"=w389) -> ("I-O.lvclass 2"=w386:refnum<class "I-O.lvclass">)  [unwired: 7 in, 1 out]
      }
      event "Secure Silicon Tray": Value Change {
        n129 = event-data() -> ()  [unwired: 1 in, 6 out]
        n130 = Index Array(array=w400, index=1) -> (element=w398:i32)
        n131 = call-dynamic "Digital Write 1 Channel.vi"("Value"=TRUE, "Channel"=w398, "I-O.lvclass"=w401) -> ("I-O.lvclass 2"=w396:refnum<class "I-O.lvclass">)  [unwired: 7 in, 1 out]
      }
      event "Go": Value Change {
        n132 = event-data() -> ()  [unwired: 1 in, 6 out]
        n133 = for {
          tunnel: "XYZTheta" -> [w416] mode=indexing
          tunnel: [w414] -> w408 mode=indexing
          shift-right: [w412] -> w407
          shift-left: w409 -> [w413]
          i -> [w418]
          n134 = Equal To 0?(x=w416) -> (x = 0?=w417:bool)
          n135 = call "Get Current Position.vi"("Gantry In"=w413) -> ("XYZTheta Out"=w411:dbl[], "Gantry Out"=w412:refnum<k24>)  [unwired: 8 in, 1 out]
          n136 = Index Array(array=w411, index=w418) -> (element=w415:dbl)
          n137 = Select(t=w415, s=w417, f=w416) -> (s? t:f=w414:dbl)
        }
        n138 = call "ClearXYZTheta Go.vi"("XYZTheta In"=w408, "Gantry In"=w407) -> ("Gantry Out"=w402:refnum<k24>)  [unwired: 7 in, 2 out]
      }
      event "Z Go": Value Change {
        n139 = event-data() -> ()  [unwired: 1 in, 6 out]
        n140 = call "Z Go.vi"("Increment"=FALSE, "Return Immediately"=FALSE ("Increment"), "Speed In"=15.0 ("Speed"), "Position In"="Position", "Gantry In"=w428) -> ("Gantry Out"=w421:refnum<k24>)  [unwired: 3 in, 3 out]
      }
      event "Stop": Value Change {
        n141 = event-data() -> ()  [unwired: 1 in, 5 out]
        n142 = call "Joystick.vi"("Joystick"=FALSE, "Gantry In"=w436) -> ("Gantry Out"=w429:refnum<k24>)  [unwired: 8 in, 1 out]
      }
    }
  }
  n143 = Bundle By Name(cluster=w1, "Gantry"=w4, "I-O.lvclass"=w3) -> (w2:T7)
  n144 = Build Array(w7, w6, w8) -> (w12:dbl[][])
  n145 = call "Release Control Cluster.vi"("output cluster"=w2) -> ()  [unwired: 11 in]
  n146 = Transpose Matrix(1:w12) -> (0:w11:dbl[][])
  n147 = Open/Create/Replace File(operation (0:open)=T6."create") -> (refnum out=w10:refnum<file>)  [unwired: 5 in, 2 out]
  n148 = Array To Spreadsheet String(array=w11, 3:"%f" ("format string")) -> (spreadsheet string=w14:string)  [unwired: 1 in]
  n149 = Write to Text File(file (use dialog)=w10, text=w14) -> (refnum out=w13:refnum<file>)  [unwired: 2 in, 2 out]
  n150 = Close File(refnum=w13) -> ()  [unwired: 1 in, 2 out]
